vi "solar Msg Voyager (TLM).vi"(8 "error in (no error)":errorcluster, 9 "TLM_DATA (No HDR)":variant, 10 "TLM":string, 11 "solar in":refnum<class "solar.lvclass">) -> (0 "error out":errorcluster, 3 "solar out":refnum<class "solar.lvclass">)   [LabVIEW 2018]
doc: "This sends telemetry back to COSMOS. If the packet is not registered with Voyager this does nothing.\n\nIf the packet name is not given, the data's label is used."
uses:
  solar.lvclass
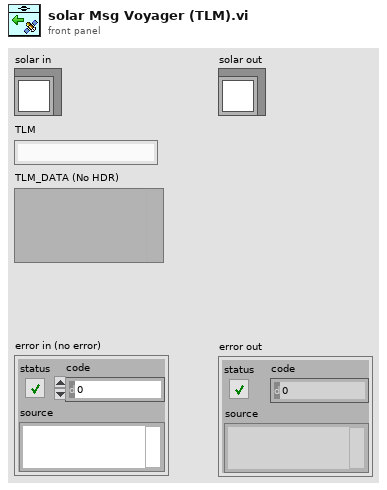
[diagram p1: front panel]
types:
  T1 = typedef "solar_voy_ctl Voyager Refnum.ctl" = refnum<k1>
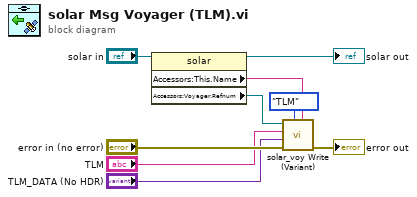
[diagram p0: block diagram]
diagram:
  n1 = property class="solar"(reference="solar in") -> (reference out=→"solar out":refnum<class "solar.lvclass">, "Accessors:This.Name"=w1:string, "Accessors:Voyager.Refnum"=w7:T1)  [unwired: 1 in, 1 out]
  n2 = call "solar_voy Write (Variant).vi"("TARGET"=w1, "CMD"=enum8{"CMD", "TLM"}."TLM", "error in (no error)"="error in (no error)", "Variant (No HDR)"="TLM_DATA (No HDR)", "PACKET (\"\" = Use Variant)"="TLM", "Voyager Refnum in"=w7) -> ("error out"=→"error out":errorcluster)  [unwired: 4 in, 1 out]
